vi "Init.vi"(8 "error in (no error)":errorcluster, 11 "VISA resource name":refnum<visa-resource-name>) -> (0 "error out":errorcluster, 3 "VISA resource out":refnum<visa-resource-name>)   [LabVIEW 2020, in "Mock Temperature Controller.lvlib"]
uses:
  Mock Temperature Controller.lvlib
  Typedefs/Init.vi States.ctl
panel:
  in  "VISA Resource":string(combo)
  in  "Connect Btn":bool
  # "The selections given are 'Mock COM Ports' they do not reflect the actual COM ports on your device"
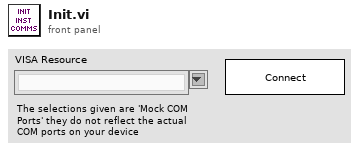
[diagram p1: front panel]
types:
  T1 = typedef "Mock Temperature Controller.lvlib/Init.vi States.ctl" = enum16{"Waiting for connection", "Connecting", "Successful connection", "Failed to connect", "Closing"}
  T2 = enum32{"Invalid", "Standard", "Closed", "Hidden", "Minimized", "Maximized"}
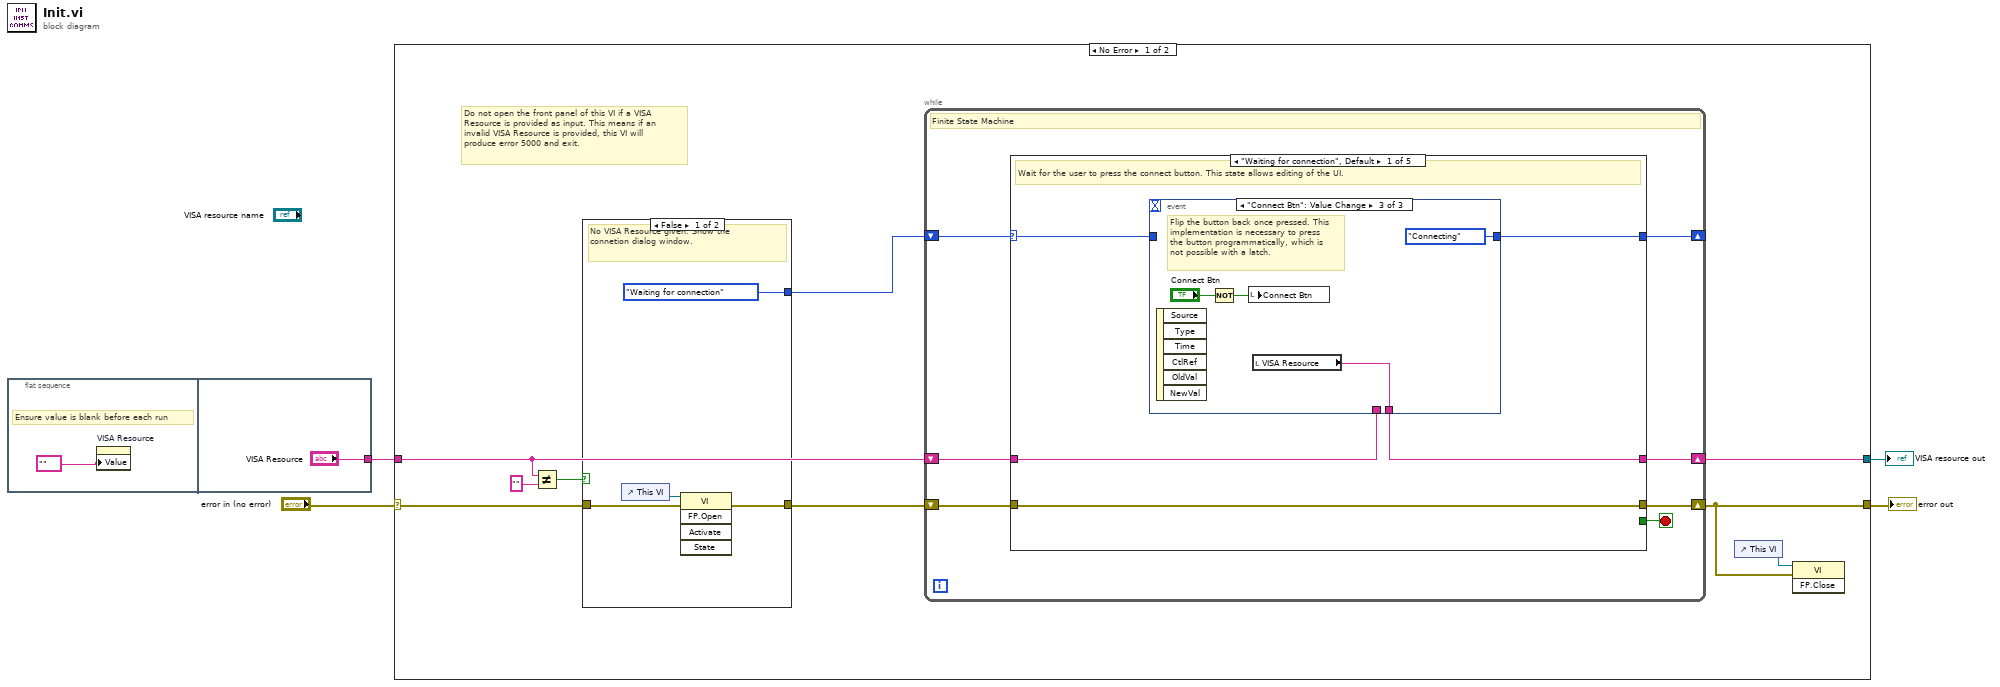
[diagram p0: block diagram]
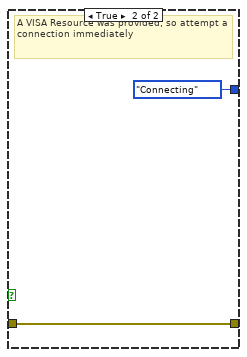
[diagram p2: hidden frame]
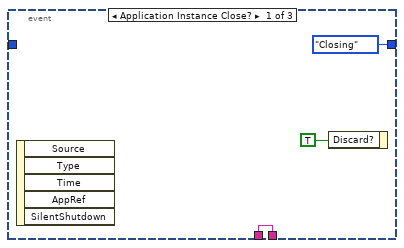
[diagram p3: hidden frame]
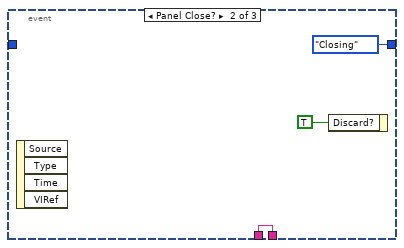
[diagram p4: hidden frame]
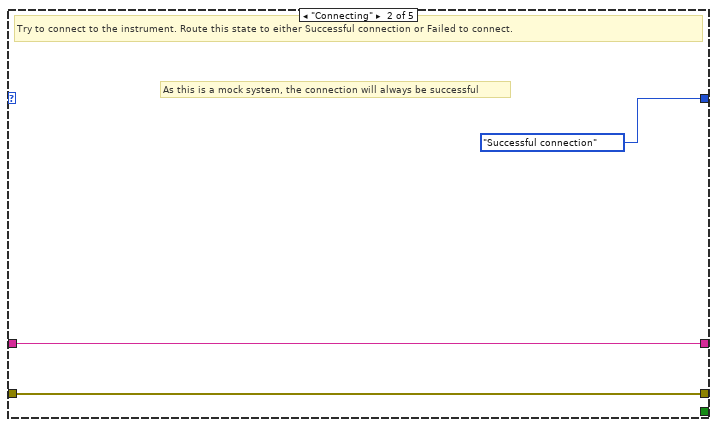
[diagram p5: hidden frame]
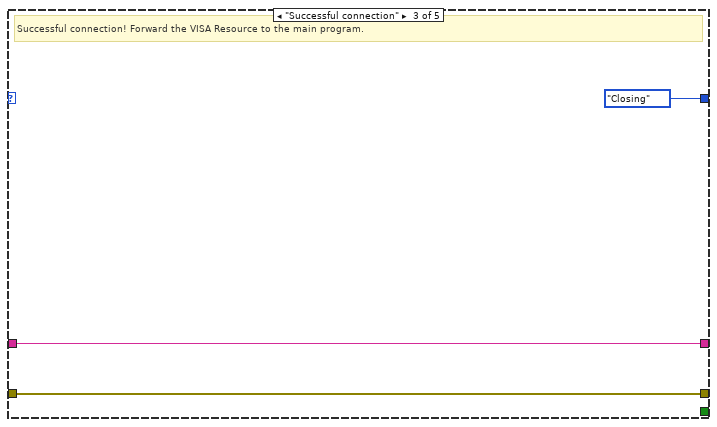
[diagram p6: hidden frame]
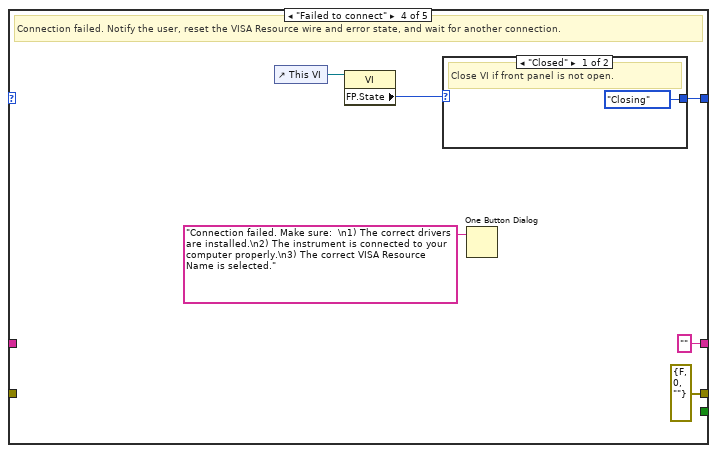
[diagram p7: hidden frame]
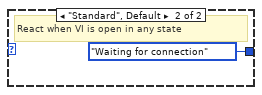
[diagram p8: hidden frame]
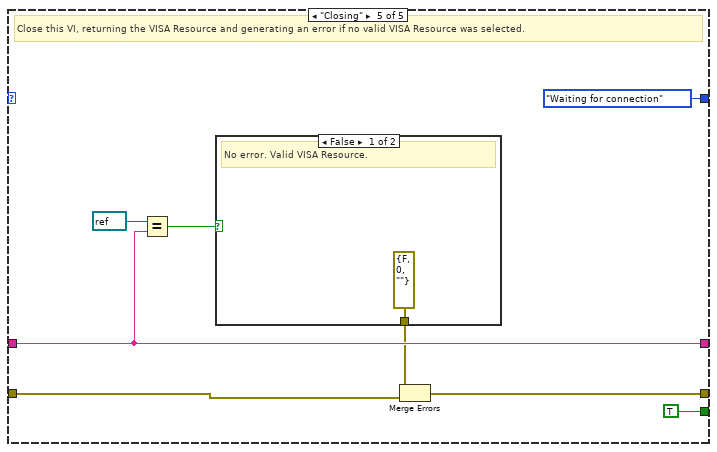
[diagram p9: hidden frame]
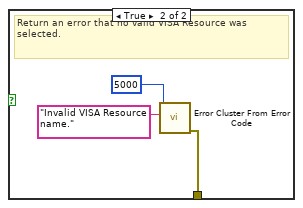
[diagram p10: hidden frame]
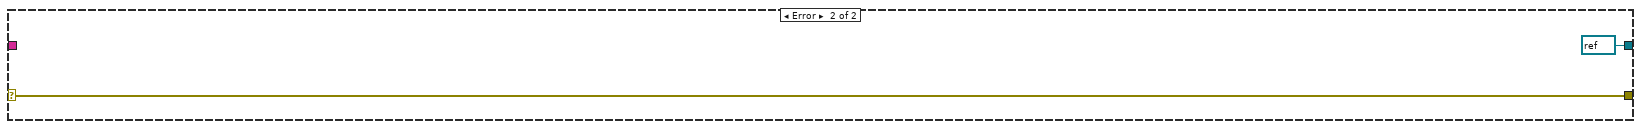
[diagram p11: hidden frame]
diagram:
  n1 = flat-sequence {
    tunnel: ["VISA Resource"] -> w1
    frame #0 {
      # "Ensure value is blank before each run"
      n2 = property on="VISA Resource" class="CmbBox"("Value"="" ("VISA Resource/Comm Port")) -> ()  [unwired: 2 in, 2 out]
    }
    frame #1 {
    }
  }
  n3 = case shown="No Error" "error in (no error)" {
    selector: "error in (no error)" -> [w10 w71]
    tunnel: [w15 refnum<visa-resource-name> refnum ("VISA resource in")] -> w4
    tunnel: [w13 w71] -> w2
    tunnel: w1 -> [w11 _]
    frame No Error {
      # "Do not open the front panel of this VI if a VISA Resource is provided as input. This means if an invalid VISA Resource is provided, this VI will produce error 5000 and exit."
      n4 = Not Equal?(x=w11, y="") -> (x != y?=w12:bool)
      n5 = case shown="False" w12 {
        tunnel: w10 -> [w18 w21]
        tunnel: [w17 w21] -> w9
        tunnel: [Init.vi_States."Waiting for connection" Init.vi_States."Connecting"] -> w8
        frame False {
          # "No VISA Resource given. Show the connetion dialog window."
          n6 = control-ref of="This VI"() -> (w19:refnum<vi>)
          n7 = invoke class="VI" method="FP.Open"(reference=w19, error in=w18) -> (error out=w17:errorcluster)  [unwired: 3 in, 4 out]
        }
        frame True {
          # "A VISA Resource was provided, so attempt a connection immediately"
        }
      }
      n8 = while {
        shift-right: [w27] -> _
        shift-left: w8 -> [w28]
        shift-right: [w25] -> w15
        shift-left: w11 -> [w24]
        shift-right: [w22] -> w13
        shift-left: w9 -> [w23]
        stop <- w26 stop-if-true
        # "Finite State Machine"
        n9 = case shown="\"Waiting for connection\", Default" w28 {
          selector: w28 -> [w33 _ _ _ _]
          tunnel: [w32 Init.vi_States."Successful connection" Init.vi_States."Closing" w55 Init.vi_States."Waiting for connection"] -> w27
          tunnel: [_ _ _ _ TRUE] -> w26
          tunnel: [w29 w45 w48 "" ("VISA Resource/Comm Port") w62] -> w25
          tunnel: w24 -> [w30 w45 w48 _ w62]
          tunnel: w23 -> [w31 w46 w47 _ w58]
          tunnel: [w31 w46 w47 errorcluster {"status"=FALSE, "code"=0, "source"=""} ("error IO") w59] -> w22
          frame "Waiting for connection", Default {
            # "Wait for the user to press the connect button. This state allows editing of the UI."
            n10 = event shown="[2] \"Connect Btn\": Value Change" {
              selector: _ -> [_ _ _]
              dyn-events: _ -> [_ _ _]
              timeout: _ -> [_ _ _]
              tunnel: [Init.vi_States."Closing" Init.vi_States."Closing" Init.vi_States."Connecting"] -> w32
              tunnel: w33 -> [_ _ _]
              tunnel: w30 -> [w34 w37 _]
              tunnel: [w34 w37 w40] -> w29
              event Application Instance Close? {
                n11 = event-data() -> ()  [unwired: 1 in, 5 out]
                n12 = event-data("Discard?"=TRUE) -> ()  [unwired: 1 in, 1 out]
              }
              event Panel Close? {
                n13 = event-data() -> ()  [unwired: 1 in, 4 out]
                n14 = event-data("Discard?"=TRUE) -> ()  [unwired: 1 in, 1 out]
              }
              event "Connect Btn": Value Change {
                # "Flip the button back once pressed. This implementation is necessary to press the button programmatically, which is not possible with a latch."
                n15 = event-data() -> ()  [unwired: 1 in, 6 out]
                n16 = Not(x="Connect Btn") -> (.not. x?=w41:bool)
                n17 = local write "Connect Btn"(w41) -> ()
                n18 = local read "VISA Resource"() -> (w40:string)
              }
            }
          }
          frame "Connecting" {
            # "As this is a mock system, the connection will always be successful"
            # "Try to connect to the instrument. Route this state to either Successful connection or Failed to connect."
          }
          frame "Successful connection" {
            # "Successful connection! Forward the VISA Resource to the main program."
          }
          frame "Failed to connect" {
            # "Connection failed. Notify the user, reset the VISA Resource wire and error state, and wait for another connection."
            n19 = control-ref of="This VI"() -> (w53:refnum<vi>)
            n20 = property class="VI"(reference=w53) -> ("FP.State"=w52:T2)  [unwired: 1 in, 2 out]
            n21 = case shown="\"Closed\"" w52 {
              tunnel: [Init.vi_States."Closing" Init.vi_States."Waiting for connection"] -> w55
              frame "Closed" {
                # "Close VI if front panel is not open."
              }
              frame "Standard", Default {
                # "React when VI is open in any state"
              }
            }
            n22 = One Button Dialog(message="Connection failed. Make sure:  \n1) The correct drivers are installed.\n2) The instrument is connected to your computer properly.\n3) The correct VISA Resource Name is selected.") -> ()  [unwired: 1 in, 1 out]
          }
          frame "Closing" {
            # "Close this VI, returning the VISA Resource and generating an error if no valid VISA Resource was selected."
            n23 = Equal?(x=refnum<visa-resource-name> refnum ("VISA resource in"), y=w62) -> (x = y?=w61:bool)
            n24 = case shown="False" w61 {
              tunnel: [errorcluster {"status"=FALSE, "code"=0, "source"=""} ("error out") w68] -> w60
              frame False {
                # "No error. Valid VISA Resource."
              }
              frame True {
                # "Return an error that no valid VISA Resource was selected."
                n25 = call <vilib>:"Error Cluster From Error Code.vi"("error message (\"\")"="Invalid VISA Resource name." ("error message (\"\")"), "error code (0)"=5000) -> ("error out"=w68:errorcluster)  [unwired: 7 in]
              }
            }
            n26 = Merge Errors(w60, w58) -> (w59:errorcluster)
          }
        }
      }
      n27 = control-ref of="This VI"() -> (w14:refnum<vi>)
      n28 = invoke class="VI" method="FP.Close"(reference=w14, error in=w13) -> ()  [unwired: 1 in, 3 out]
    }
    frame Error {
    }
  }
  "VISA resource out" <- w4
  "error out" <- w2
